vi "Format Data to Image.vi"(10 "# B-lines":i32, 11 "data in":sgl[](array[numeric])) -> (2 "float data":sgl[][][](array[numeric]), 3 "U16bit data":u16[][][](array[numeric]))   [LabVIEW 2018]
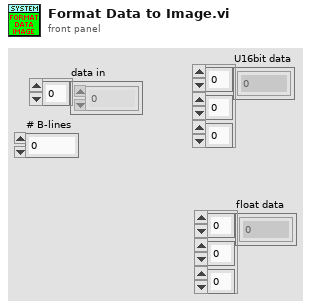
[diagram p1: front panel]
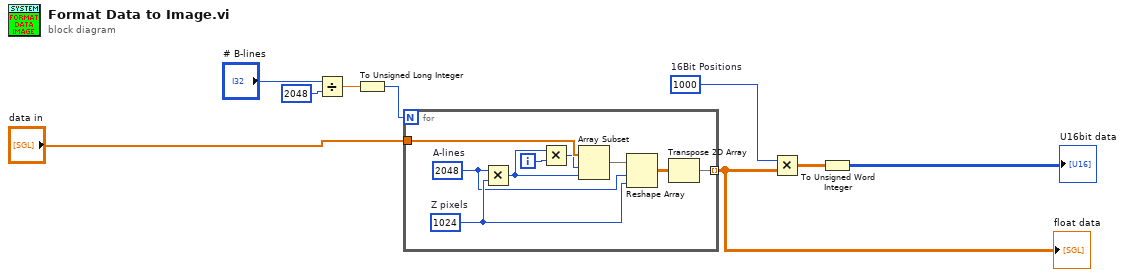
[diagram p0: block diagram]
diagram:
  w5 = 1000  # 16Bit Positions
  n1 = Divide(x="# B-lines", y=2048) -> (x/y=w2:dbl)
  n2 = To Unsigned Long Integer(number=w2) -> (unsigned 32bit integer=w1:u32)
  n3 = for {
    N: w1 -> [_]
    tunnel: "data in" -> [w15]
    tunnel: [w13] -> w7 mode=indexing
    i -> [w12]
    w17 = 1024  # Z pixels
    w16 = 2048  # A-lines
    n4 = Multiply(x=w16, y=w17) -> (x*y=w11:i32)
    n5 = Multiply(x=w11, y=w12) -> (x*y=w10:i32)
    n6 = Array Subset(array=w15, index=w10, length=w11) -> (w18:sgl[])
    n7 = Reshape Array(w18, w16, w17) -> (w14:sgl[][])
    n8 = Transpose 2D Array(2D array=w14) -> (transposed array=w13:sgl[][])
  }
  "float data" <- w7
  n9 = Multiply(x=w5, y=w7) -> (x*y=w6:sgl[][][])
  n10 = To Unsigned Word Integer(number=w6) -> (unsigned 16bit integer=→"U16bit data":u16[][][])
